vi "BER.vi"(11 "Confusion Matrix":i32[][](array[numeric])) -> (3 "BER":dbl)   [LabVIEW 2019]
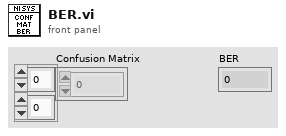
[diagram p1: front panel]
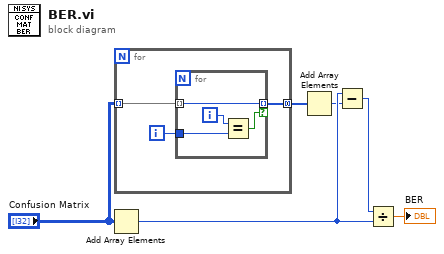
[diagram p0: block diagram]
diagram:
  n1 = Add Array Elements(numeric array="Confusion Matrix") -> (sum=w5:i32)
  n2 = for {
    tunnel: "Confusion Matrix" -> [w8] mode=indexing
    tunnel: [w7] -> w1 mode=concatenating
    i -> [w9]
    n3 = for {
      tunnel: w9 -> [w13]
      tunnel: w8 -> [w11] mode=indexing
      tunnel: [w11] -> w7 mode=indexing if=w10
      i -> [w12]
      n4 = Equal?(x=w12, y=w13) -> (x = y?=w10:bool)
    }
  }
  n5 = Add Array Elements(numeric array=w1) -> (sum=w3:i32)
  n6 = Subtract(x=w5, y=w3) -> (x-y=w4:i32)
  n7 = Divide(x=w4, y=w5) -> (x/y=→"BER":dbl)
